vi "Main.vi"(8 "error in (no error)":errorcluster, 11 "StageSPIMBase in":refnum<class "StageSPIM.lvclass">) -> (0 "error out":errorcluster, 3 "component":refnum<class "StageSPIM.lvclass">)   [LabVIEW 2012, in "StageSPIM.lvclass"]
doc: "Main VI of the component."
uses:
  StageSPIM.lvclass
  <vilib>/Distrio/Murmex/Murmex/command_enum.ctl
  StageSPIM.lvclass/StageSPIM.ctl
  <vilib>/Distrio/Murmex/InitialiseMessage/InitialiseMessage.lvclass
  <vilib>/Distrio/Murmex/GenericMessage/GenericMessage.lvclass
  <vilib>/Distrio/Murmex/TerminateMessage/TerminateMessage.lvclass
  <vilib>/Distrio/Murmex/Murmex/update_cluster.ctl
  <vilib>/Distrio/Murmex/StopMessage/StopMessage.lvclass
  <vilib>/Distrio/Murmex/ConfigureMessage/ConfigureMessage.lvclass
  <vilib>/Distrio/Murmex/Murmex/Set configure at initialise.vi
  <vilib>/Distrio/Murmex/Murmex/Set log reference.vi
  <vilib>/Distrio/Murmex/Murmex/Set VI reference.vi
  <vilib>/Distrio/Murmex/Murmex/Get ID.vi
  <vilib>/Distrio/Murmex/Murmex/Murmex.lvclass
  <vilib>/Distrio/Murmex/Message/Message.lvclass
panel:
  in  "button::stop":bool
  in  "button::configure":bool
  in  "button::quit":bool
  in  "Tab Control":enum32{"Main", "Debug"}(tab)
  in  "forwardY":bool
  in  "backY":bool
  in  "stepY":dbl[unit]
  in  "forwardZ":bool
  in  "backZ":bool
  in  "stepZ":dbl[unit]
  in  "forwardX":bool
  in  "backX":bool
  in  "stepX":dbl[unit]
  in  "forwardA":bool
  in  "backA":bool
  in  "stepA":dbl[unit]
  out "currentA":dbl[unit]
  out "currentX":dbl[unit]
  out "currentY":dbl[unit]
  out "currentZ":dbl[unit]
  in  "speedZ":dbl[unit]
  in  "speedY":dbl[unit]
  in  "speedX":dbl[unit]
  in  "speedA":dbl[unit]
  in  "targetA":dbl[unit]
  in  "targetX":dbl[unit]
  in  "targetY":dbl[unit]
  in  "targetZ":dbl[unit]
  in  "button::send":bool
  out "log":string
  in  "command":T1
  in  "Generic command":string
  in  "ID":string="stage"
  out "terminate?":bool=TRUE
  # "Current\nposition"
  # "Target\nposition"
  # "Steps"
  # "Speed"
  # "A"
  # "X"
  # "Y"
  # "Z"
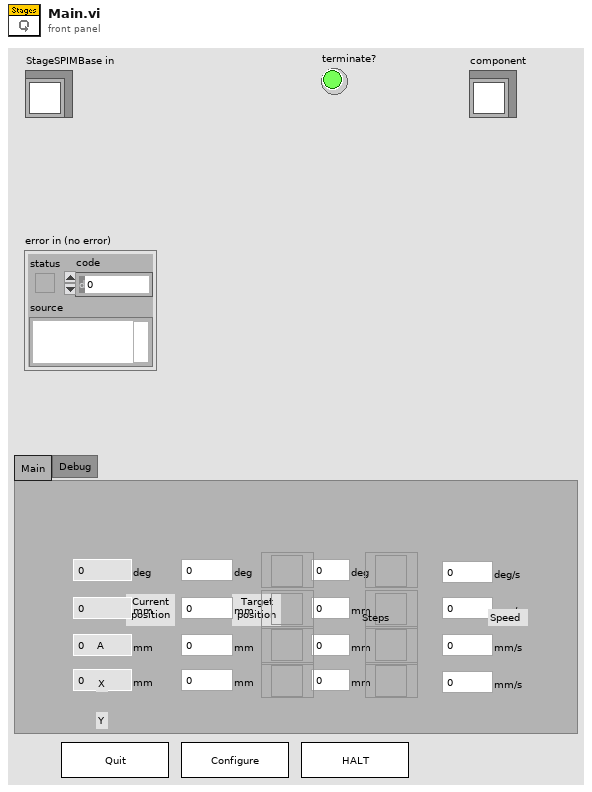
[diagram p1: front panel]
types:
  T1 = typedef "Murmex.lvlib/Murmex.lvclass/command_enum.ctl" = enum16{"null", "initialise", "reset", "terminate", "acknowledge", "update", "inspect", "inform", "proceed", "start", "stop", "fetch", "configure", "generic"}
  T2 = enum8{"Enabled", "Disabled", "Disabled and Grayed Out"}
  T3 = typedef "Murmex.lvlib/Murmex.lvclass/update_cluster.ctl" = cluster{"target ID":string, "key chains":string[], "values":variant[]}
  T4 = typedef "Murmex.lvlib/Murmex.lvclass/Event type enumerations.ctl" = enum16{"before", "after"}
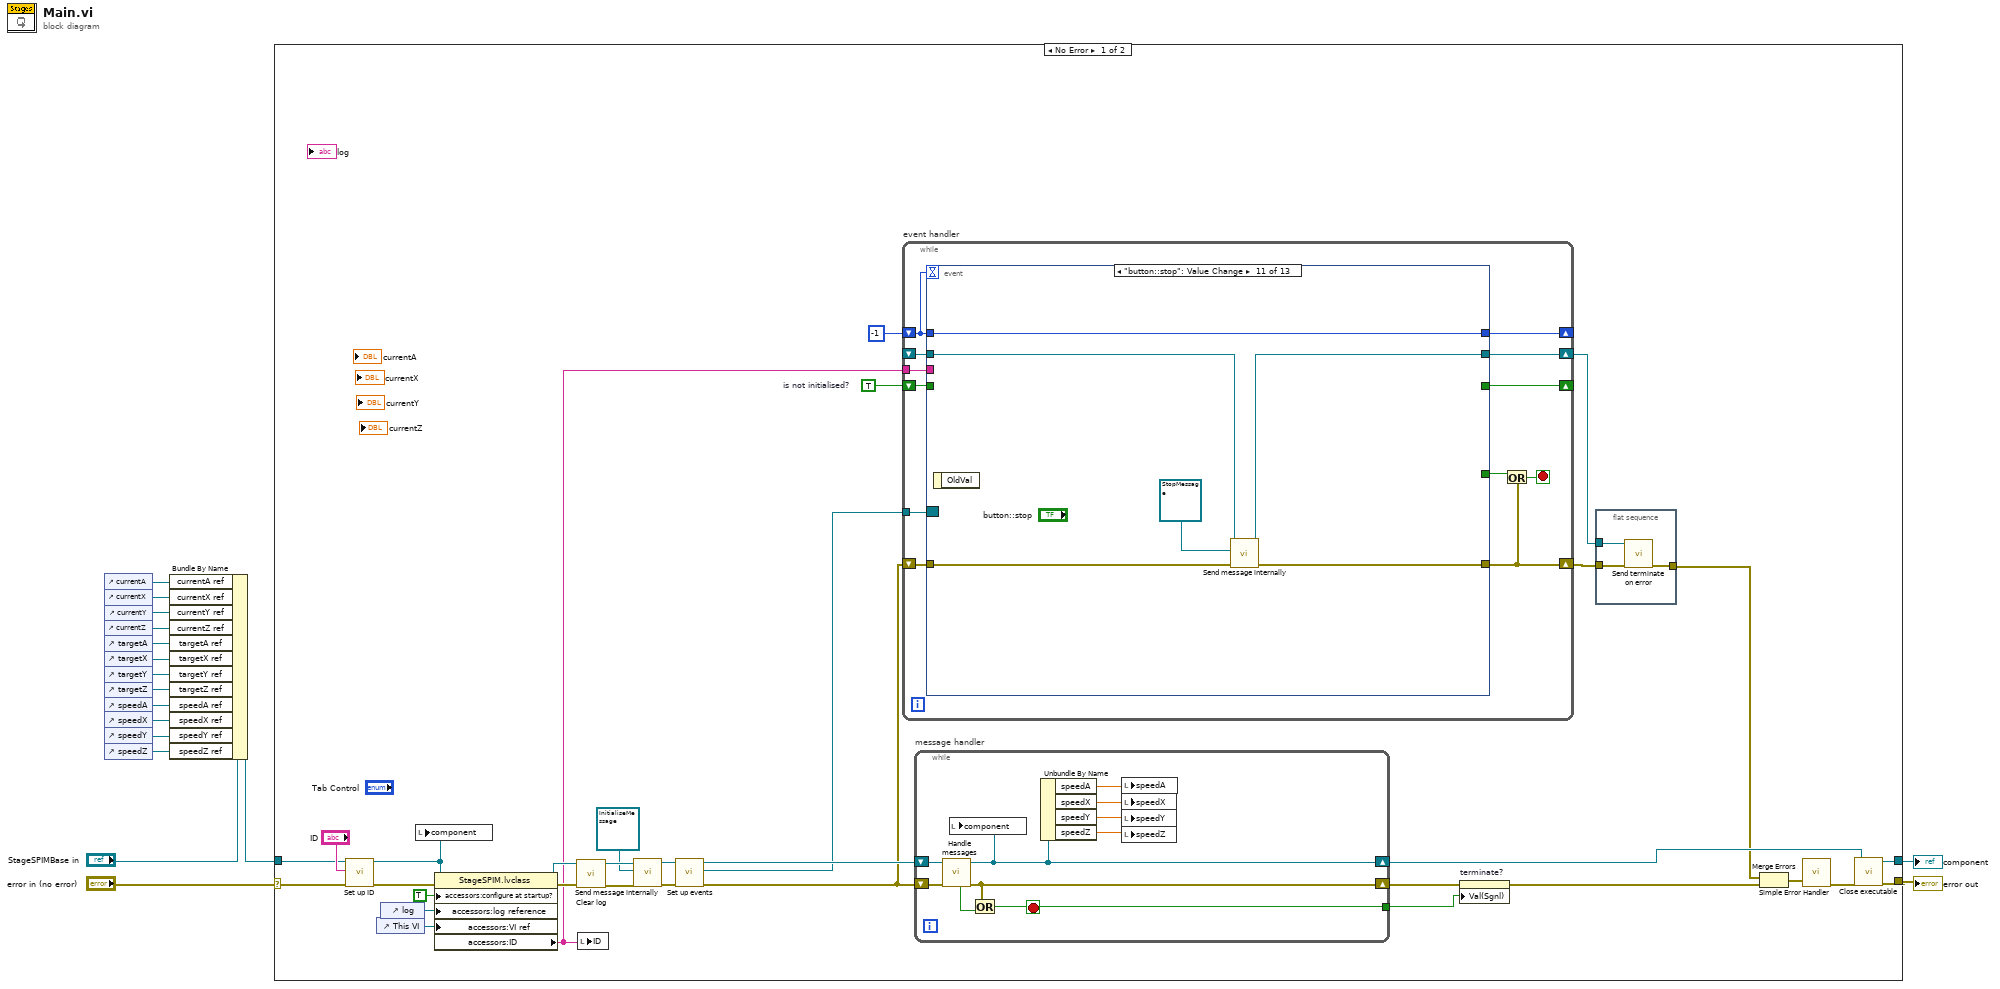
[diagram p0: block diagram]
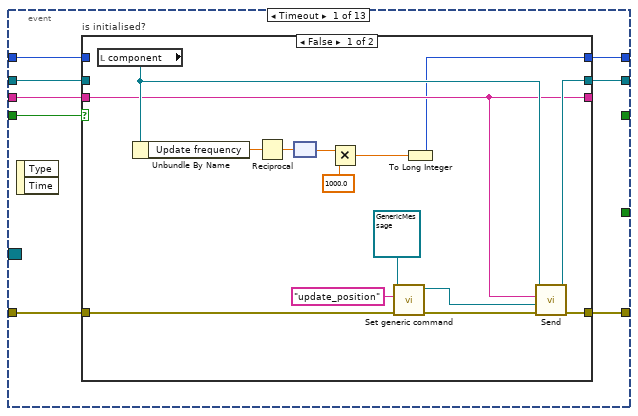
[diagram p2: hidden frame]
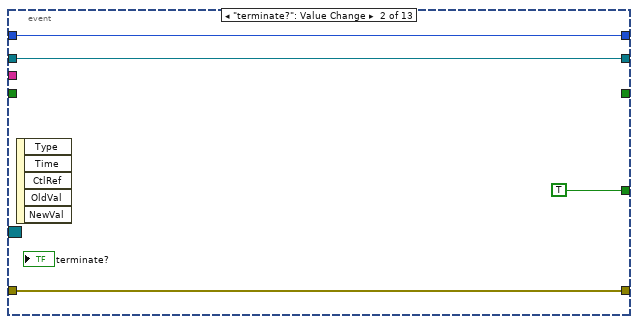
[diagram p4: hidden frame]
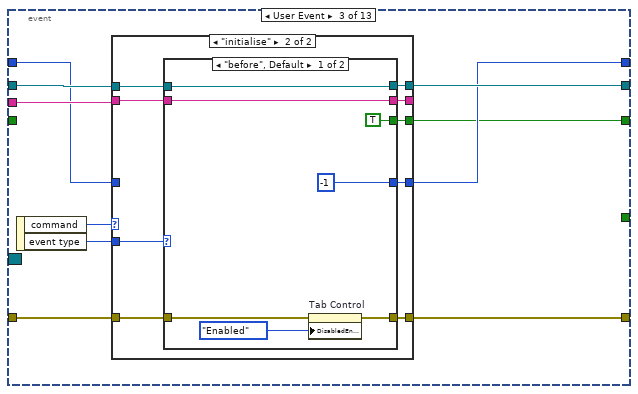
[diagram p5: hidden frame]
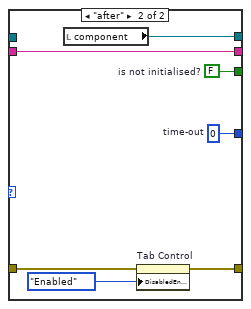
[diagram p7: hidden frame]
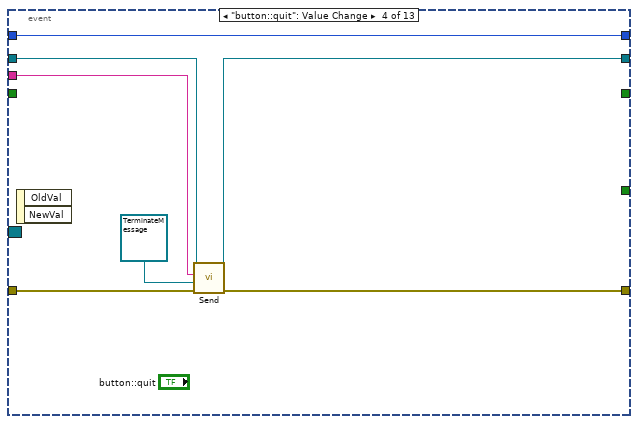
[diagram p8: hidden frame]
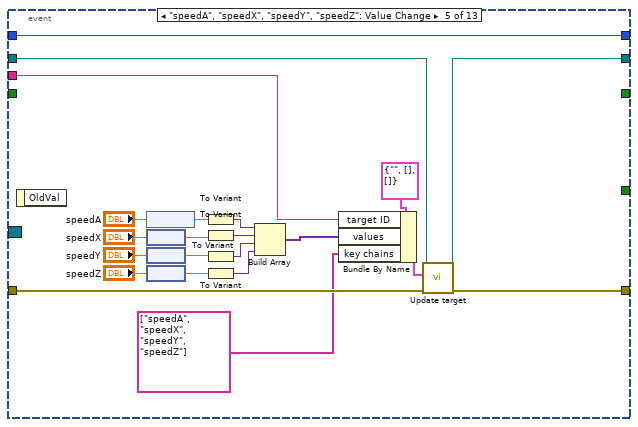
[diagram p9: hidden frame]
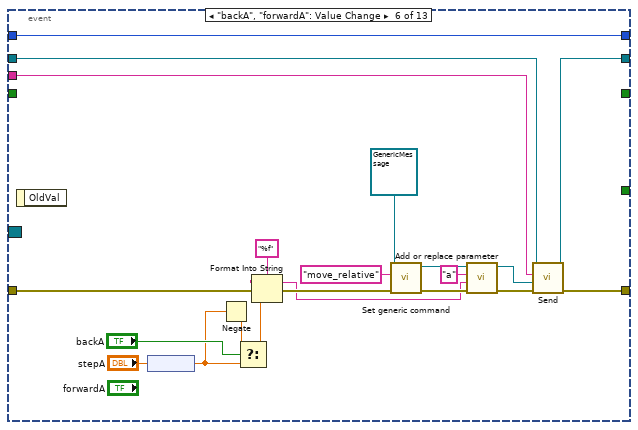
[diagram p10: hidden frame]
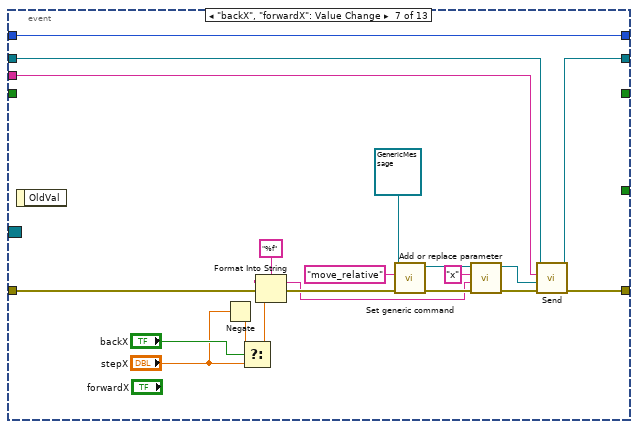
[diagram p11: hidden frame]
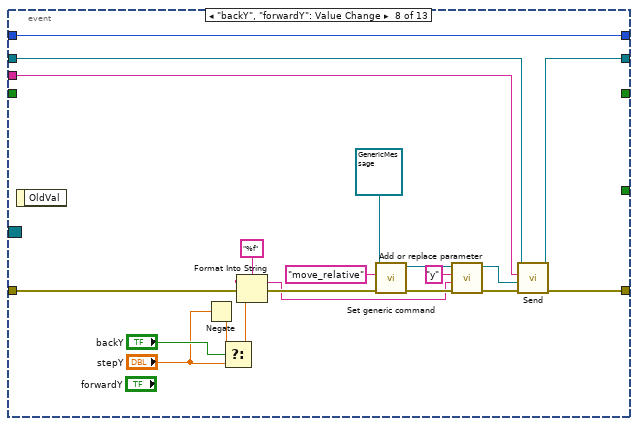
[diagram p12: hidden frame]
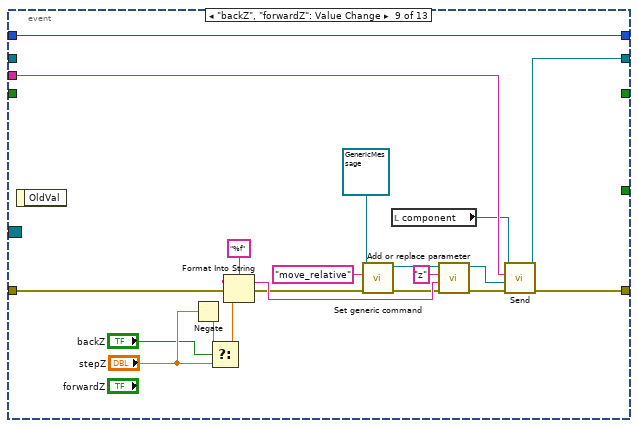
[diagram p13: hidden frame]
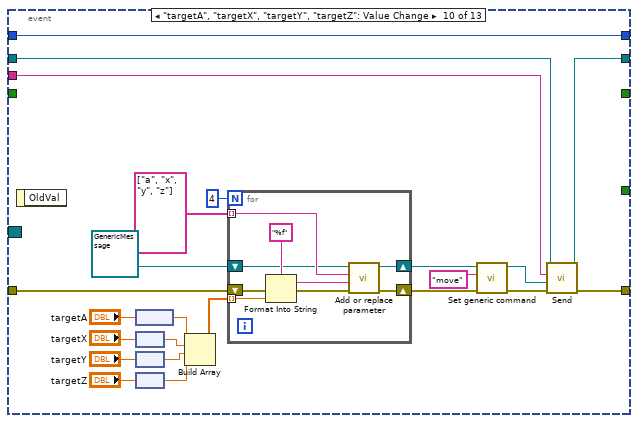
[diagram p14: hidden frame]
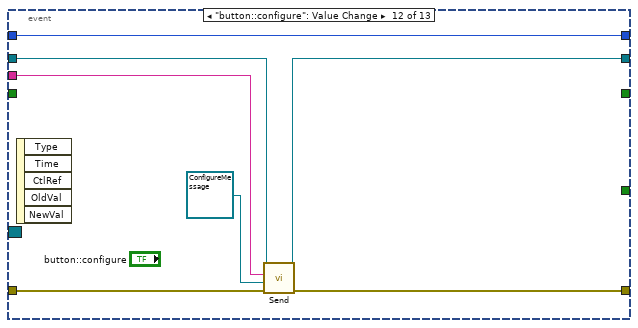
[diagram p15: hidden frame]
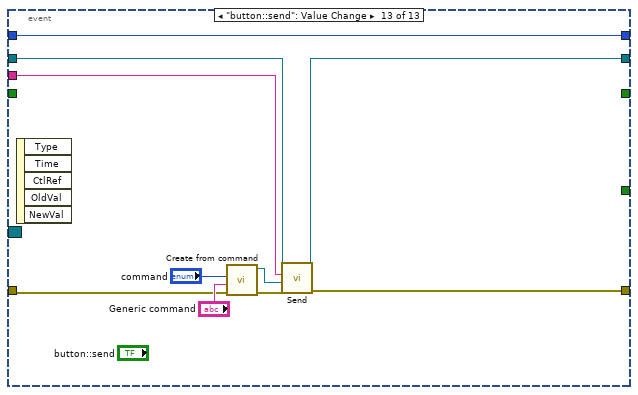
[diagram p16: hidden frame]
diagram:
  n1 = control-ref of="currentA"() -> (w12:refnum<vi>)
  n2 = control-ref of="currentX"() -> (w11:refnum<vi>)
  n3 = control-ref of="currentY"() -> (w10:refnum<vi>)
  n4 = control-ref of="currentZ"() -> (w9:refnum<vi>)
  n5 = control-ref of="targetA"() -> (w8:refnum<vi>)
  n6 = control-ref of="targetX"() -> (w7:refnum<vi>)
  n7 = control-ref of="targetY"() -> (w6:refnum<vi>)
  n8 = control-ref of="targetZ"() -> (w5:refnum<vi>)
  n9 = control-ref of="speedA"() -> (w4:refnum<vi>)
  n10 = control-ref of="speedX"() -> (w3:refnum<vi>)
  n11 = control-ref of="speedY"() -> (w2:refnum<vi>)
  n12 = control-ref of="speedZ"() -> (w1:refnum<vi>)
  n13 = Bundle By Name(cluster="StageSPIMBase in", "currentA ref"=w12, "currentX ref"=w11, "currentY ref"=w10, "currentZ ref"=w9, "targetA ref"=w8, "targetX ref"=w7, "targetY ref"=w6, "targetZ ref"=w5, "speedA ref"=w4, "speedX ref"=w3, "speedY ref"=w2, "speedZ ref"=w1) -> (w15:refnum<class "StageSPIM.lvclass">)
  n14 = case shown="No Error" "error in (no error)" {
    selector: "error in (no error)" -> [w48 w308]
    tunnel: w15 -> [w47 w309]
    tunnel: [w32 w308] -> w14
    tunnel: [w30 w309] -> w13
    frame No Error {
      w22 = TRUE  # is not initialised?
      n15 = call <vilib>:"Set up ID.vi"("error in (no error)"=w48, "component ID"="ID", "MurmexBase in"=w47) -> ("error out"=w46:errorcluster, "MurmexBase out"=w23:refnum<class "StageSPIM.lvclass">)  [unwired: 6 in, 1 out]
      n16 = control-ref of="This VI"() -> (w43:refnum<vi>)
      n17 = control-ref of="log"() -> (w44:refnum<vi>)
      n18 = local write "component"(w23) -> ()
      n19 = property class="StageSPIM.lvclass"(reference=w23, error in=w46, "accessors:configure at startup?"=TRUE ("configure at startup?"), "accessors:log reference"=w44, "accessors:VI ref"=w43) -> (reference out=w41:refnum<class "StageSPIM.lvclass">, error out=w42:errorcluster, "accessors:ID"=w24:string)
      n20 = call <vilib>:"Clear log.vi"("error in (no error)"=w42, "MurmexBase in"=w41) -> ("error out"=w40:errorcluster, "MurmexBase out"=w39:refnum<class "StageSPIM.lvclass">)  [unwired: 8 in]
      n21 = local write "ID"(w24) -> ()
      n22 = call <vilib>:"Send message internally.vi"("error in (no error)"=w40, "Message"=refnum<class "InitialiseMessage.lvclass"> refnum ("Distrio Murmex 1.1:InitialiseMessage"), "Murmex in"=w39) -> ("error out"=w37:errorcluster, "Murmex out"=w36:refnum<class "StageSPIM.lvclass">)  [unwired: 7 in]
      n23 = call <vilib>:"Set up events.vi"("error in (no error)"=w37, "MurmexBase in"=w36) -> ("error out"=w29:errorcluster, "Event Registration Refnum"=w28:refnum<event-registration>, "MurmexBase out"=w35:refnum<class "StageSPIM.lvclass">)  [unwired: 7 in]
      n24 = while "event handler" {
        shift-right: [w55] -> w26
        shift-left: w29 -> [w64]
        tunnel: w28 -> [w63]
        shift-right: [w61] -> _
        shift-left: -1 -> [w62]
        shift-right: [w58] -> w18
        shift-left: _ -> [w57]
        shift-right: [w53] -> _
        shift-left: w22 -> [w54]
        tunnel: w24 -> [w59]
        stop <- w60 stop-if-true
        n25 = event shown="[10] \"button::stop\": Value Change" {
          selector: w63 -> [_ _ _ _ _ _ _ _ _ _ _ _ _]
          dyn-events: _ -> [_ _ _ _ _ _ _ _ _ _ _ _ _]
          timeout: w62 -> [_ _ _ _ _ _ _ _ _ _ _ _ _]
          tunnel: w64 -> [w71 w95 w105 w138 w159 w181 w184 w206 w226 w243 w280 w287 w293]
          tunnel: w62 -> [w65 w93 w97 w133 w144 w182 w183 w205 w227 w260 w278 w281 w289]
          tunnel: [w72 w93 w98 w133 w144 w182 w183 w205 w227 w260 w278 w281 w289] -> w61
          tunnel: [w70 w95 w99 w137 w158 w171 w190 w210 w229 w264 w276 w286 w292] -> w55
          tunnel: w59 -> [w69 _ w102 w134 w157 w168 w187 w207 w228 w261 _ w284 w288]
          tunnel: w57 -> [w67 w92 w101 w136 w156 w170 w188 w208 _ w262 w279 w283 w291]
          tunnel: [w68 w92 w100 w135 w155 w169 w189 w209 w230 w263 w277 w282 w290] -> w58
          tunnel: [_ TRUE _ _ _ _ _ _ _ _ _ _ _] -> w56
          tunnel: w54 -> [w66 _ _ _ _ _ _ _ _ _ _ _ _]
          tunnel: [_ _ w96 _ _ _ _ _ _ _ _ _ _] -> w53
          event Timeout {
            n26 = event-data() -> ()  [unwired: 1 in, 2 out]
            n27 = case "is initialised?" shown="False" w66 {
              tunnel: [w73 w88] -> w72
              tunnel: w71 -> [w81 w91]
              tunnel: [w80 w91] -> w70
              tunnel: w69 -> [w76 w90]
              tunnel: [w78 w89] -> w68
              tunnel: w67 -> [_ w89]
              tunnel: [w76 w90] -> _
              tunnel: w65 -> [_ w88]
              frame False {
                n28 = local read "component"() -> (w77:refnum<class "StageSPIM.lvclass">)
                n29 = Unbundle By Name(w77) -> ("Update frequency"=w87:dbl[unit])
                n30 = Reciprocal(x=w87) -> (1/x=w86:dbl[unit])
                n31 = node(w86) -> (w75:dbl)
                n32 = Multiply(x=w75, y=1000.0) -> (x*y=w74:dbl)
                n33 = call <vilib>:"Set generic command.vi"("error in (no error)"=w81, "generic command"="update_position", "GenericMessage in"=refnum<class "GenericMessage.lvclass"> refnum ("Distrio Murmex 1.1:GenericMessage")) -> ("error out"=w82:errorcluster, "GenericMessage out"=w79:refnum<class "GenericMessage.lvclass">)  [unwired: 7 in]
                n34 = To Long Integer(number=w74) -> (32bit integer=w73:i32)
                n35 = call <vilib>:"Send.vi"("error in (no error)"=w82, "Message"=w79, "recipient"=w76, "Murmex in"=w77) -> ("error out"=w80:errorcluster, "Murmex out"=w78:refnum<class "StageSPIM.lvclass">)  [unwired: 6 in]
              }
              frame True {
              }
            }
          }
          event "terminate?": Value Change {
            n36 = event-data() -> ()  [unwired: 1 in, 5 out]
          }
          event User Event {
            n37 = event-data() -> ("command"=w104:T1, "event type"=w103:T4)  [unwired: 1 in]
            n38 = case shown="\"initialise\"" w104 {
              tunnel: w105 -> [w107 w118]
              tunnel: [w107 w117] -> w99
              tunnel: w102 -> [w109 w116]
              tunnel: [w108 w115] -> w100
              tunnel: w101 -> [w108 w114]
              tunnel: [w109 w113] -> _
              tunnel: w103 -> [_ w112]
              tunnel: [w106 w111] -> w98
              tunnel: w97 -> [w106 _]
              tunnel: [_ w110] -> w96
              frame "null", Default {
              }
              frame "initialise" {
                n39 = case shown="\"before\", Default" w112 {
                  tunnel: [w124 w131] -> w117
                  tunnel: w118 -> [w125 w132]
                  tunnel: w116 -> [w122 w128]
                  tunnel: [w121 w130] -> w115
                  tunnel: w114 -> [w121 _]
                  tunnel: [w122 w128] -> w113
                  tunnel: [-1 w127] -> w111
                  tunnel: [TRUE ("is not initialised?") w126] -> w110
                  frame "before", Default {
                    n40 = property on="Tab Control" class="TabCtl (strict)"(error in=w125, "DisabledEnum"=T2."Enabled" ("Disabled")) -> (error out=w124:errorcluster)  [unwired: 1 in, 1 out]
                  }
                  frame "after" {
                    w126 = FALSE  # is not initialised?
                    w127 = 0  # time-out
                    n41 = local read "component"() -> (w130:refnum<class "StageSPIM.lvclass">)
                    n42 = property on="Tab Control" class="TabCtl (strict)"(error in=w132, "DisabledEnum"=T2."Enabled" ("Disabled")) -> (error out=w131:errorcluster)  [unwired: 1 in, 1 out]
                  }
                }
              }
            }
          }
          event "button::quit": Value Change {
            n43 = event-data() -> ()  [unwired: 1 in, 2 out]
            n44 = call <vilib>:"Send.vi"("error in (no error)"=w138, "Message"=refnum<class "TerminateMessage.lvclass"> refnum ("Murmex.lvlib:TerminateMessage"), "recipient"=w134, "Murmex in"=w136) -> ("error out"=w137:errorcluster, "Murmex out"=w135:refnum<class "StageSPIM.lvclass">)  [unwired: 6 in]
          }
          event "speedA", "speedX", "speedY", "speedZ": Value Change {
            n45 = event-data() -> ()  [unwired: 1 in, 1 out]
            n46 = node("speedA") -> (w143:dbl)
            n47 = node("speedX") -> (w140:dbl)
            n48 = node("speedY") -> (w141:dbl)
            n49 = node("speedZ") -> (w142:dbl)
            n50 = To Variant(anything=w143) -> (Variant=w150:variant)
            n51 = To Variant(anything=w140) -> (Variant=w149:variant)
            n52 = To Variant(anything=w141) -> (Variant=w148:variant)
            n53 = To Variant(anything=w142) -> (Variant=w147:variant)
            n54 = Build Array(w150, w149, w148, w147) -> (w146:variant[])
            n55 = Bundle By Name(cluster=T3 {"target ID"="", "key chains"=[], "values"=[]} ("update cluster"), "target ID"=w157, "values"=w146, "key chains"=string[] ["speedA", "speedX", "speedY", "speedZ"]) -> (w161:T3)
            n56 = call <vilib>:"Update target.vi"("error in (no error)"=w159, "update cluster"=w161, "MurmexBase in"=w156) -> ("error out"=w158:errorcluster, "MurmexBase out"=w155:refnum<class "StageSPIM.lvclass">)  [unwired: 7 in]
          }
          event "backA", "forwardA": Value Change {
            n57 = event-data() -> ()  [unwired: 1 in, 1 out]
            n58 = node("stepA") -> (w162:dbl)
            n59 = Negate(x=w162) -> (-x=w175:dbl)
            n60 = Select(t=w175, s="backA", f=w162) -> (s? t:f=w164:dbl)
            n61 = Format Into String(format string="%f", error in=w181, w164) -> (resulting string=w165:string, error out=w172:errorcluster)  [unwired: 1 in]
            n62 = call <vilib>:"Set generic command.vi"("error in (no error)"=w172, "generic command"="move_relative", "GenericMessage in"=refnum<class "GenericMessage.lvclass"> refnum ("Distrio Murmex 1.1:GenericMessage")) -> ("error out"=w179:errorcluster, "GenericMessage out"=w177:refnum<class "GenericMessage.lvclass">)  [unwired: 7 in]
            n63 = call <vilib>:"Add or replace parameter.vi"("error in (no error)"=w179, "value"=w165, "name"="a", "Message in"=w177) -> ("error out"=w178:errorcluster, "Message out"=w166:refnum<class "GenericMessage.lvclass">)  [unwired: 6 in]
            n64 = call <vilib>:"Send.vi"("error in (no error)"=w178, "Message"=w166, "recipient"=w168, "Murmex in"=w170) -> ("error out"=w171:errorcluster, "Murmex out"=w169:refnum<class "StageSPIM.lvclass">)  [unwired: 6 in]
          }
          event "backX", "forwardX": Value Change {
            n65 = event-data() -> ()  [unwired: 1 in, 1 out]
            n66 = Negate(x="stepX") -> (-x=w197:dbl[unit])
            n67 = Select(t=w197, s="backX", f="stepX") -> (s? t:f=w192:dbl[unit])
            n68 = Format Into String(format string="%f", error in=w184, w192) -> (resulting string=w193:string, error out=w196:errorcluster)  [unwired: 1 in]
            n69 = call <vilib>:"Set generic command.vi"("error in (no error)"=w196, "generic command"="move_relative", "GenericMessage in"=refnum<class "GenericMessage.lvclass"> refnum ("Distrio Murmex 1.1:GenericMessage")) -> ("error out"=w201:errorcluster, "GenericMessage out"=w199:refnum<class "GenericMessage.lvclass">)  [unwired: 7 in]
            n70 = call <vilib>:"Add or replace parameter.vi"("error in (no error)"=w201, "value"=w193, "name"="x", "Message in"=w199) -> ("error out"=w200:errorcluster, "Message out"=w194:refnum<class "GenericMessage.lvclass">)  [unwired: 6 in]
            n71 = call <vilib>:"Send.vi"("error in (no error)"=w200, "Message"=w194, "recipient"=w187, "Murmex in"=w188) -> ("error out"=w190:errorcluster, "Murmex out"=w189:refnum<class "StageSPIM.lvclass">)  [unwired: 6 in]
          }
          event "backY", "forwardY": Value Change {
            n72 = event-data() -> ()  [unwired: 1 in, 1 out]
            n73 = Negate(x="stepY") -> (-x=w217:dbl[unit])
            n74 = Select(t=w217, s="backY", f="stepY") -> (s? t:f=w212:dbl[unit])
            n75 = Format Into String(format string="%f", error in=w206, w212) -> (resulting string=w213:string, error out=w216:errorcluster)  [unwired: 1 in]
            n76 = call <vilib>:"Set generic command.vi"("error in (no error)"=w216, "generic command"="move_relative", "GenericMessage in"=refnum<class "GenericMessage.lvclass"> refnum ("Distrio Murmex 1.1:GenericMessage")) -> ("error out"=w221:errorcluster, "GenericMessage out"=w219:refnum<class "GenericMessage.lvclass">)  [unwired: 7 in]
            n77 = call <vilib>:"Add or replace parameter.vi"("error in (no error)"=w221, "value"=w213, "name"="y", "Message in"=w219) -> ("error out"=w220:errorcluster, "Message out"=w214:refnum<class "GenericMessage.lvclass">)  [unwired: 6 in]
            n78 = call <vilib>:"Send.vi"("error in (no error)"=w220, "Message"=w214, "recipient"=w207, "Murmex in"=w208) -> ("error out"=w210:errorcluster, "Murmex out"=w209:refnum<class "StageSPIM.lvclass">)  [unwired: 6 in]
          }
          event "backZ", "forwardZ": Value Change {
            n79 = event-data() -> ()  [unwired: 1 in, 1 out]
            n80 = Negate(x="stepZ") -> (-x=w236:dbl[unit])
            n81 = Select(t=w236, s="backZ", f="stepZ") -> (s? t:f=w241:dbl[unit])
            n82 = Format Into String(format string="%f", error in=w226, w241) -> (resulting string=w240:string, error out=w237:errorcluster)  [unwired: 1 in]
            n83 = call <vilib>:"Set generic command.vi"("error in (no error)"=w237, "generic command"="move_relative", "GenericMessage in"=refnum<class "GenericMessage.lvclass"> refnum ("Distrio Murmex 1.1:GenericMessage")) -> ("error out"=w232:errorcluster, "GenericMessage out"=w234:refnum<class "GenericMessage.lvclass">)  [unwired: 7 in]
            n84 = local read "component"() -> (w223:refnum<class "StageSPIM.lvclass">)
            n85 = call <vilib>:"Add or replace parameter.vi"("error in (no error)"=w232, "value"=w240, "name"="z", "Message in"=w234) -> ("error out"=w233:errorcluster, "Message out"=w239:refnum<class "GenericMessage.lvclass">)  [unwired: 6 in]
            n86 = call <vilib>:"Send.vi"("error in (no error)"=w233, "Message"=w239, "recipient"=w228, "Murmex in"=w223) -> ("error out"=w229:errorcluster, "Murmex out"=w230:refnum<class "StageSPIM.lvclass">)  [unwired: 6 in]
          }
          event "targetA", "targetX", "targetY", "targetZ": Value Change {
            n87 = event-data() -> ()  [unwired: 1 in, 1 out]
            n88 = node("targetA") -> (w246:dbl)
            n89 = node("targetX") -> (w251:dbl)
            n90 = node("targetY") -> (w247:dbl)
            n91 = node("targetZ") -> (w248:dbl)
            n92 = Build Array(w246, w251, w247, w248) -> (w244:dbl[])
            n93 = for {
              N: 4 -> [_]
              shift-right: [w272] -> w257
              shift-left: w243 -> [w271]
              tunnel: string[] ["a", "x", "y", "z"] -> [w270] mode=indexing
              shift-right: [w268] -> w253
              shift-left: refnum<class "GenericMessage.lvclass"> refnum ("Distrio Murmex 1.1:GenericMessage") -> [w269]
              tunnel: w244 -> [w267] mode=indexing
              n94 = Format Into String(format string="%f", error in=w271, w267) -> (resulting string=w266:string, error out=w273:errorcluster)  [unwired: 1 in]
              n95 = call <vilib>:"Add or replace parameter.vi"("error in (no error)"=w273, "value"=w266, "name"=w270, "Message in"=w269) -> ("error out"=w272:errorcluster, "Message out"=w268:refnum<class "GenericMessage.lvclass">)  [unwired: 6 in]
            }
            n96 = call <vilib>:"Set generic command.vi"("error in (no error)"=w257, "generic command"="move", "GenericMessage in"=w253) -> ("error out"=w259:errorcluster, "GenericMessage out"=w258:refnum<class "GenericMessage.lvclass">)  [unwired: 7 in]
            n97 = call <vilib>:"Send.vi"("error in (no error)"=w259, "Message"=w258, "recipient"=w261, "Murmex in"=w262) -> ("error out"=w264:errorcluster, "Murmex out"=w263:refnum<class "StageSPIM.lvclass">)  [unwired: 6 in]
          }
          event "button::stop": Value Change {
            n98 = event-data() -> ()  [unwired: 1 in, 1 out]
            n99 = call <vilib>:"Send message internally.vi"("error in (no error)"=w280, "Message"=refnum<class "StopMessage.lvclass"> refnum ("Distrio Murmex 1.5:StopMessage"), "Murmex in"=w279) -> ("error out"=w276:errorcluster, "Murmex out"=w277:refnum<class "StageSPIM.lvclass">)  [unwired: 7 in]
          }
          event "button::configure": Value Change {
            n100 = event-data() -> ()  [unwired: 1 in, 5 out]
            n101 = call <vilib>:"Send.vi"("error in (no error)"=w287, "Message"=refnum<class "ConfigureMessage.lvclass"> refnum ("Distrio Murmex 1.1:ConfigureMessage"), "recipient"=w284, "Murmex in"=w283) -> ("error out"=w286:errorcluster, "Murmex out"=w282:refnum<class "StageSPIM.lvclass">)  [unwired: 6 in]
          }
          event "button::send": Value Change {
            n102 = event-data() -> ()  [unwired: 1 in, 5 out]
            n103 = call <vilib>:"Create from command.vi"("error in (no error)"=w293, "generic command"="Generic command", "command"="command") -> ("error out"=w295:errorcluster, "Message out"=w296:refnum<class "Message.lvclass">)  [unwired: 7 in]
            n104 = call <vilib>:"Send.vi"("error in (no error)"=w295, "Message"=w296, "recipient"=w288, "Murmex in"=w291) -> ("error out"=w292:errorcluster, "Murmex out"=w290:refnum<class "StageSPIM.lvclass">)  [unwired: 6 in]
          }
        }
        n105 = Or(x=w56, y=w55) -> (x .or. y?=w60:bool)
      }
      n106 = while "message handler" {
        shift-right: [w305] -> w21
        shift-left: w29 -> [w307]
        shift-right: [w302] -> w31
        shift-left: w35 -> [w306]
        tunnel: [w303] -> w19
        stop <- w303 stop-if-true
        n107 = call <vilib>:"Handle messages.vi"("error in (no error)"=w307, "Murmex in"=w306) -> ("error out"=w305:errorcluster, "Murmex out"=w302:refnum<class "StageSPIM.lvclass">, "terminated?"=w304:bool)  [unwired: 7 in]
        n108 = local write "component"(w302) -> ()
        n109 = Or(x=w305, y=w304) -> (x .or. y?=w303:bool)
        n110 = Unbundle By Name(w302) -> ("speedA"=w301:dbl[unit], "speedX"=w300:dbl[unit], "speedY"=w299:dbl[unit], "speedZ"=w298:dbl[unit])
        n111 = local write "speedA"(w301) -> ()
        n112 = local write "speedX"(w300) -> ()
        n113 = local write "speedY"(w299) -> ()
        n114 = local write "speedZ"(w298) -> ()
      }
      n115 = property on="terminate?" class="Bool (strict)"(error in=w21, "Val(Sgnl)"=w19) -> (error out=w20:errorcluster)  [unwired: 1 in, 1 out]
      n116 = flat-sequence {
        tunnel: w26 -> [w52]
        tunnel: [w51] -> w25
        tunnel: w18 -> [w50]
        frame #0 {
          n117 = call <vilib>:"Send terminate on error.vi"("error in (no error)"=w52, "Murmex in"=w50) -> ("error out"=w51:errorcluster)  [unwired: 8 in, 1 out]
        }
      }
      n118 = Merge Errors(w25, w20) -> (w34:errorcluster)
      n119 = call <vilib>:"Simple Error Handler.vi"("error in (no error)"=w34) -> ("error out"=w33:errorcluster)  [unwired: 4 in, 4 out]
      n120 = call <vilib>:"Close executable.vi"("error in (no error)"=w33, "MurmexBase in"=w31) -> ("error out"=w32:errorcluster, "MurmexBase out"=w30:refnum<class "StageSPIM.lvclass">)  [unwired: 8 in]
    }
    frame Error {
    }
  }
  "error out" <- w14
  "component" <- w13
